vi "registerEvents.vi"(8 "error in (no error)":errorcluster, 11 "SAL_Listener in":refnum<class "SAL_Listener.lvclass">) -> (0 "error out":errorcluster, 3 "SAL_Listener out":refnum<class "SAL_Listener.lvclass">)   [LabVIEW 2016, in "SAL_Listener.lvclass"]
uses:
  SAL_Listener.lvclass
  SAL_Listener.lvclass/SAL_Listener.ctl
  SALLV_dome/SALLV_dome.lvlib
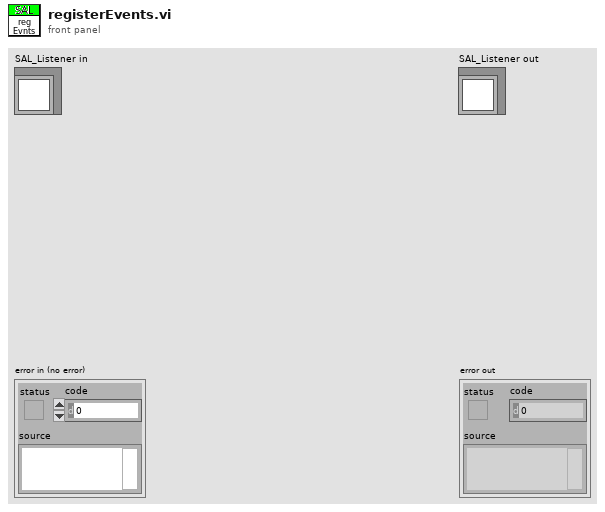
[diagram p1: front panel]
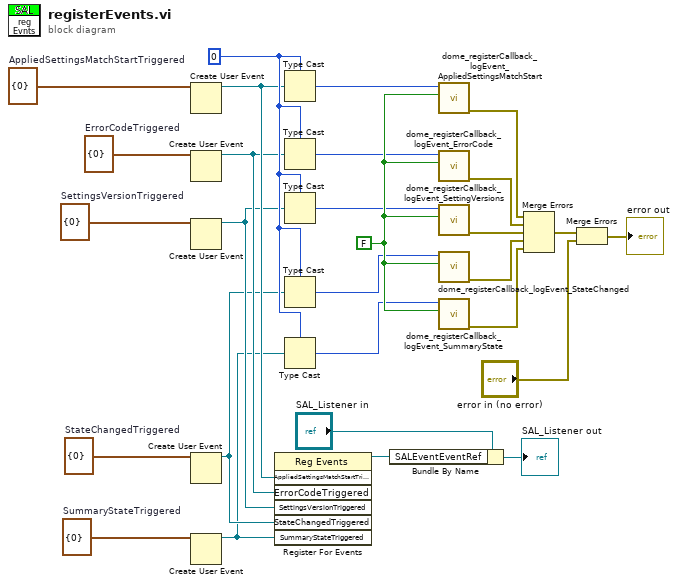
[diagram p0: block diagram]
diagram:
  w22 = cluster{"data":i32} {"data"=0}  # SummaryStateTriggered
  w23 = cluster{"data":i32} {"data"=0}  # StateChangedTriggered
  w24 = cluster{"data":i32} {"data"=0}  # SettingsVersionTriggered
  w25 = cluster{"data":i32} {"data"=0}  # ErrorCodeTriggered
  w26 = FALSE
  w17 = 0 ("handle")
  w28 = cluster{"data":i32} {"data"=0}  # AppliedSettingsMatchStartTriggered
  n1 = Create User Event(user event datatype=w28) -> (user event=w8:refnum<user-event>)  [unwired: 1 in, 1 out]
  n2 = Create User Event(user event datatype=w25) -> (user event=w7:refnum<user-event>)  [unwired: 1 in, 1 out]
  n3 = Create User Event(user event datatype=w24) -> (user event=w6:refnum<user-event>)  [unwired: 1 in, 1 out]
  n4 = Create User Event(user event datatype=w23) -> (user event=w5:refnum<user-event>)  [unwired: 1 in, 1 out]
  n5 = Create User Event(user event datatype=w22) -> (user event=w4:refnum<user-event>)  [unwired: 1 in, 1 out]
  n6 = register-events(w8, w7, w6, w5, w4) -> (reference out=w2:refnum<event-registration>)  [unwired: 2 in, 1 out]
  n7 = Type Cast(type=w17, x=w8) -> (*(type *) &x=w27:i32)
  n8 = Type Cast(type=w17, x=w7) -> (*(type *) &x=w18:i32)
  n9 = Type Cast(type=w17, x=w6) -> (*(type *) &x=w19:i32)
  n10 = Type Cast(type=w17, x=w5) -> (*(type *) &x=w20:i32)
  n11 = Type Cast(type=w17, x=w4) -> (*(type *) &x=w21:i32)
  n12 = Bundle By Name(cluster="SAL_Listener in", "SALEventEventRef"=w2) -> (→"SAL_Listener out":refnum<class "SAL_Listener.lvclass">)
  n13 = call "dome_registerCallback_logEvent_AppliedSettingsMatchStart.vi"("skipOld"=w26, "handle"=w27) -> ("error out"=w16:errorcluster)  [unwired: 8 in, 1 out]
  n14 = call "dome_registerCallback_logEvent_ErrorCode.vi"("skipOld"=w26, "handle"=w18) -> ("error out"=w15:errorcluster)  [unwired: 8 in, 1 out]
  n15 = call "dome_registerCallback_logEvent_SettingVersions.vi"("skipOld"=w26, "handle"=w19) -> ("error out"=w14:errorcluster)  [unwired: 8 in, 1 out]
  n16 = call "dome_registerCallback_logEvent_StateChanged.vi"("skipOld"=w26, "handle"=w20) -> ("error out"=w13:errorcluster)  [unwired: 8 in, 1 out]
  n17 = call "dome_registerCallback_logEvent_SummaryState.vi"("skipOld"=w26, "handle"=w21) -> ("error out"=w12:errorcluster)  [unwired: 8 in, 1 out]
  n18 = Merge Errors(w16, w15, w14, w13, w12) -> (w11:errorcluster)
  n19 = Merge Errors(w11, "error in (no error)") -> (→"error out":errorcluster)
